vi "数据查询_仪器数据.vi"() -> ()   [LabVIEW 2016, in "数据查询.lvlib"]
uses:
  <vilib>/Utility/miscctls.llb/LVPointTypeDef.ctl
  <vilib>/Utility/miscctls.llb/LVDateTimeRec.ctl
  <vilib>/Utility/miscctls.llb/LVRowAndColumnUnsignedTypeDef.ctl
  <userlib>/_OpenG.lib/array/array.llb/Sort 2D Array (String)__ogtk.vi
  <vilib>/ptbypt/NI_PtbyPt.lvlib
panel:
  out "技术要求":T1={"氨氮"=[0.2, 0.05, 0.1, 0.1], "总磷"=[0.02, 0.05, 0.1, 0.1], "总氮"=[0.3, 0.05, 0.1, 0.1], "CODMn"=[1.5, 0.1, 0.1, 0.1], "CODCr"=[5.0, 0.05, 0.1, 0.1]}
  in  "技术要求":bool
  in  "参数选择":string(combo)="全部数据"
  out "布尔":bool=TRUE
  in  "显示关键参数":bool
  in  "剔除异常数据":bool
  in  "数据类型":string(combo)="全部数据"
  in  "列表框":i32(listbox)
  in  "页":i32 format="第%.0f页"
  in  "每页条数":i32=1000
  in  "向后按钮":bool
  in  "向前按钮":bool
  in  "导出":bool
  in  "测量模式":string(combo)="全部数据"
  in  "查询":bool
  in  "结束日期":string="2050/01/01"
  in  "起始日期":string="2010/01/01"
  out "数据表":string[][](table)
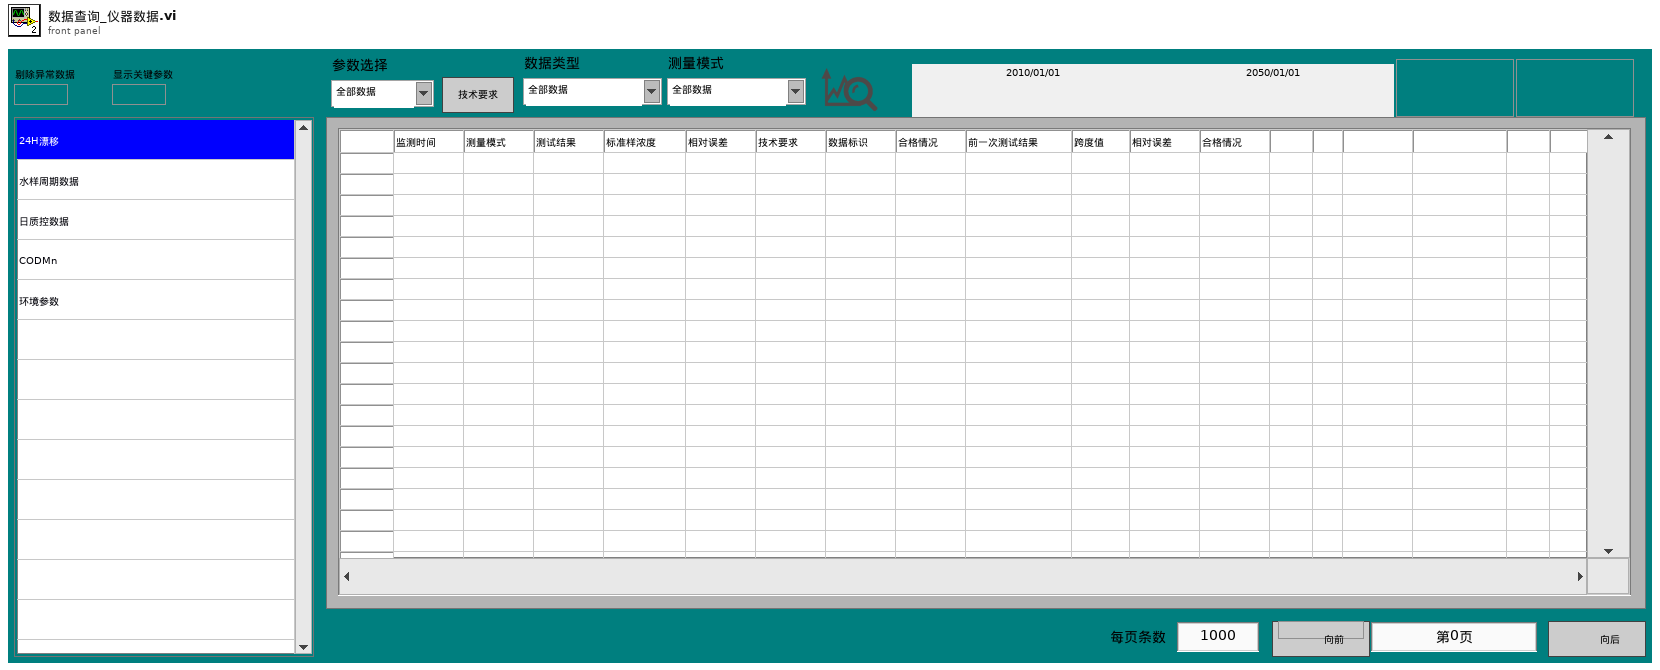
[diagram p1: front panel]
types:
  T1 = cluster{"氨氮":dbl[], "总磷":dbl[], "总氮":dbl[], "CODMn":dbl[], "CODCr":dbl[]}
  T2 = typedef "LVPointTypeDef.ctl" = cluster{"Horizontal":i16, "Vertical":i16}
  T3 = typedef "LVDateTimeRec.ctl" = cluster{"秒数的小数部分":dbl, "秒":i32, "分":i32, "时":i32, "日":i32, "月":i32, "年":i32, "天数（周）":i32, "天数（年）":i32, "DST":i32}
  T4 = typedef "Rendezvous RefNum" = refnum<k1>
  T5 = typedef "数据查询.lvlib/数据查询单选控件.ctl" = enum32{"数据查询", "仪器数据", "仪器日志", "报警信息", "校准日志"}
  T6 = enum8{"Enabled", "Disabled", "Disabled and Grayed Out"}
  T7 = cluster{"索引起始时间":timestamp, "索引终止时间":timestamp, "模式":enum16{"零点核查", "跨度核查"}, "table":string, "误差":enum16{"绝对误差", "相对误差"}, "技术要求":sgl, "24H漂移技术要求":sgl}
  T8 = typedef "LVRowAndColumnUnsignedTypeDef.ctl" = cluster{"Row":u32, "Column":u32}
  T9 = typedef "数据库类型.ctl" = enum16{"Access", "SQLite"}
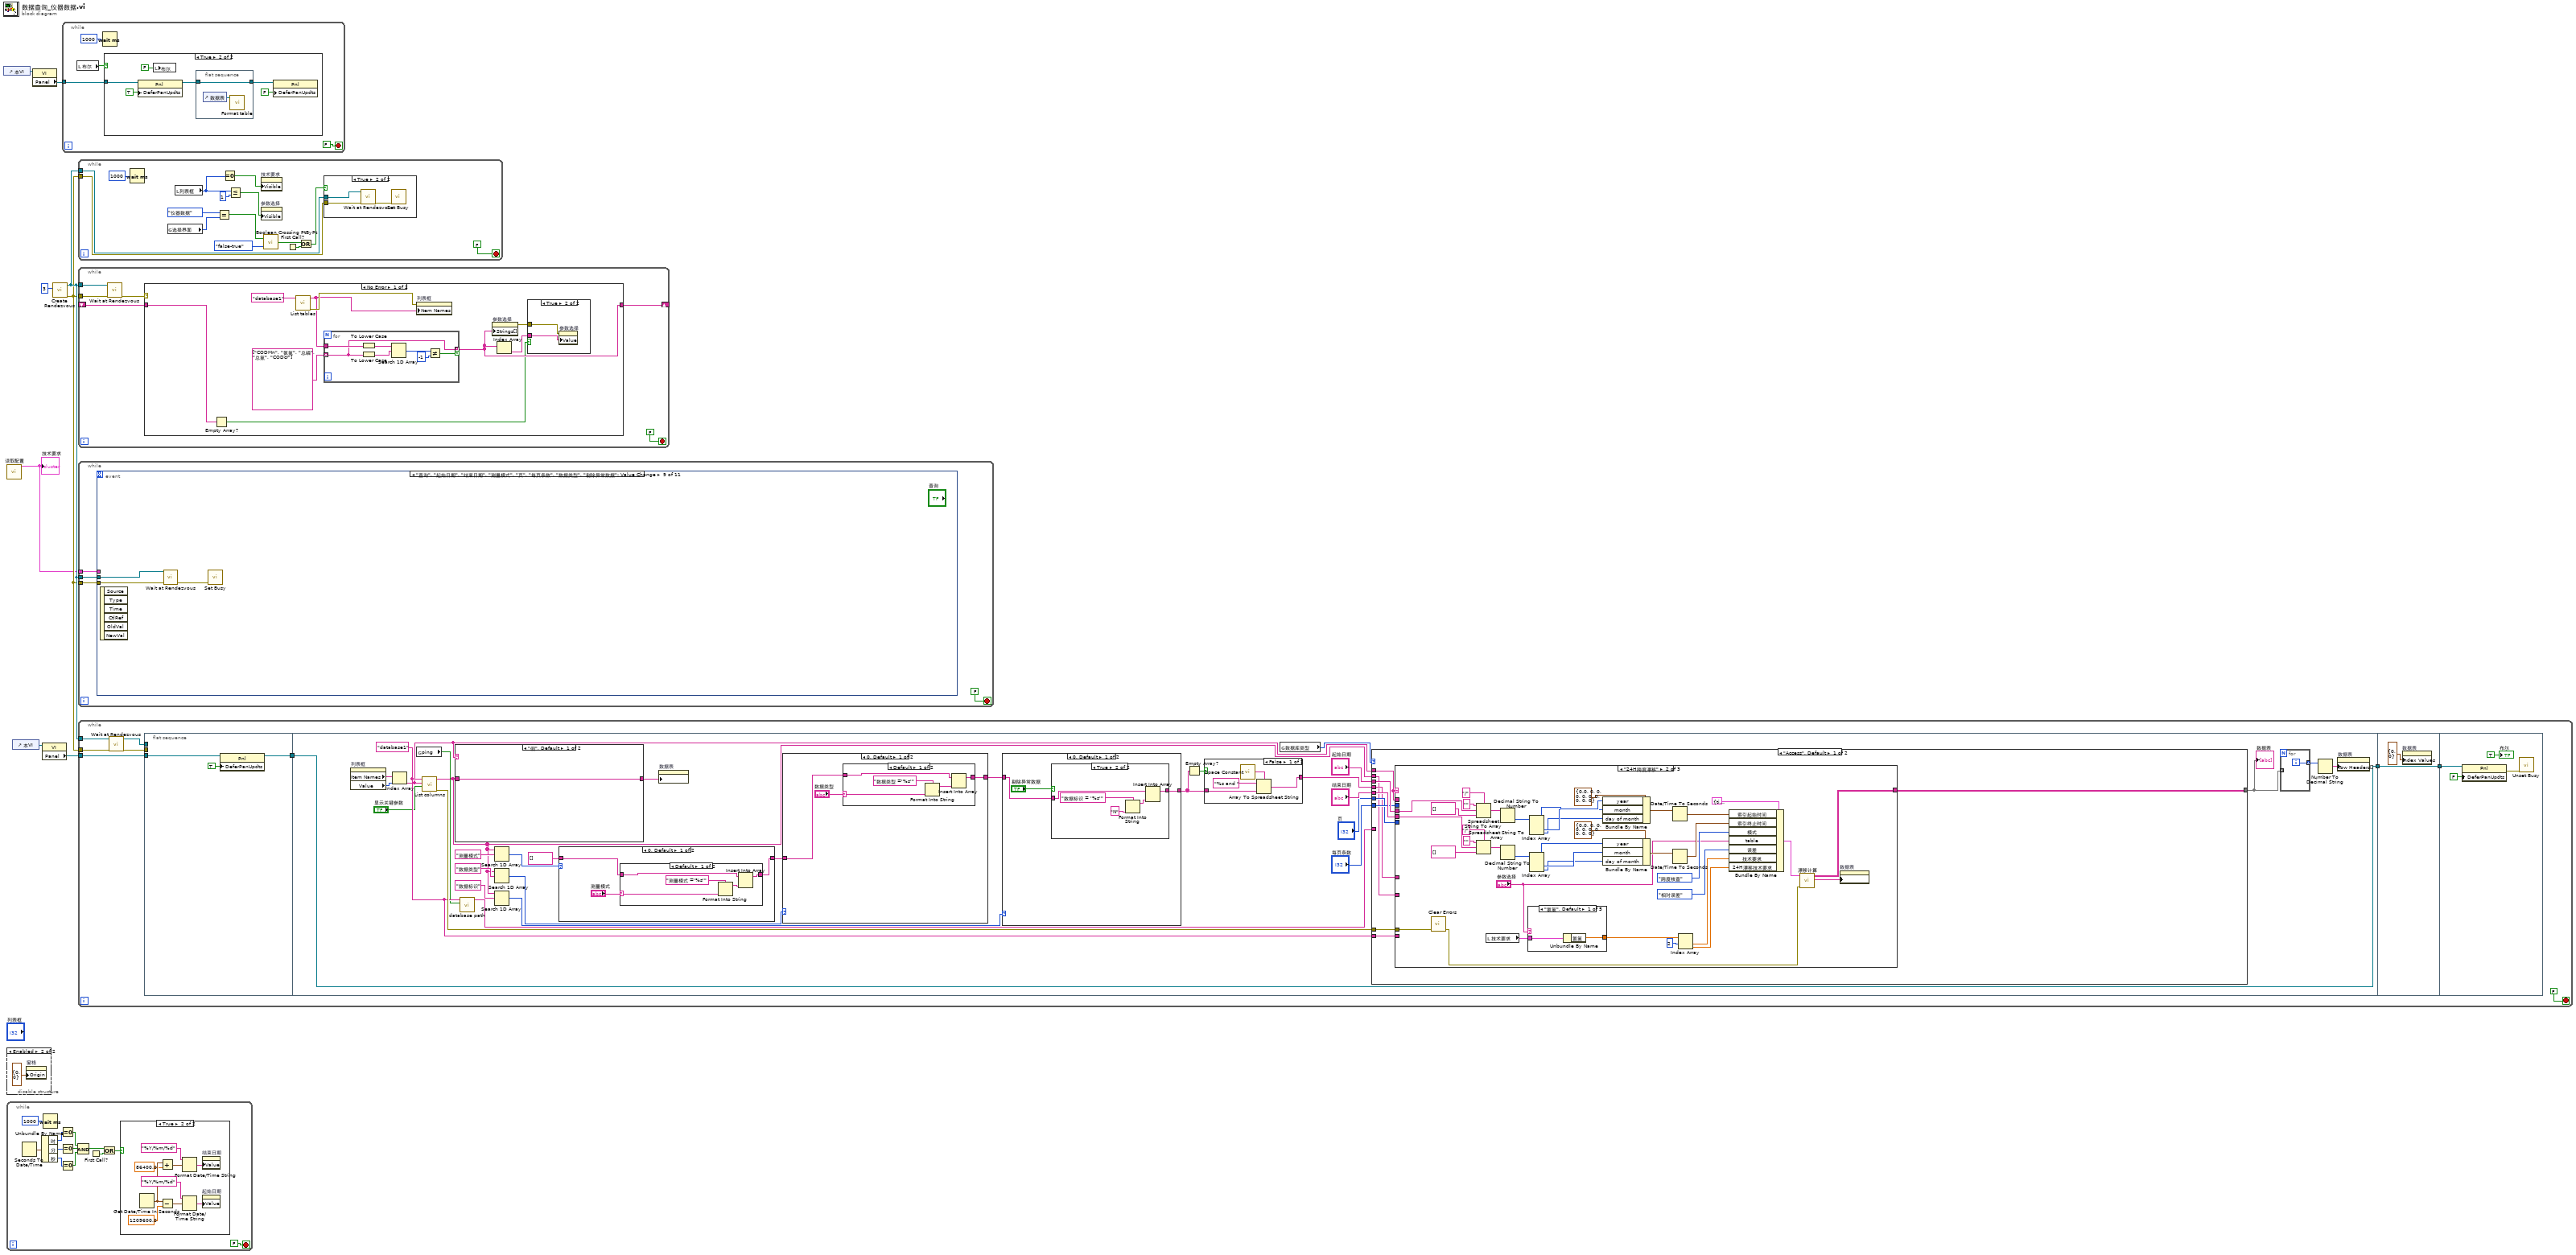
[diagram p0: block diagram]
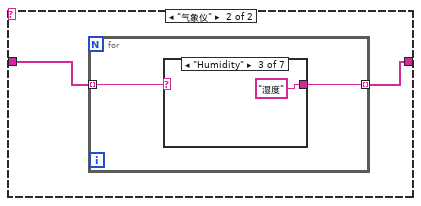
[diagram p6: hidden frame]
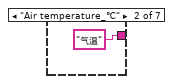
[diagram p8: hidden frame]
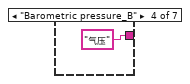
[diagram p9: hidden frame]
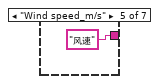
[diagram p10: hidden frame]
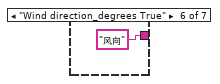
[diagram p11: hidden frame]
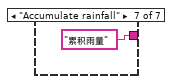
[diagram p12: hidden frame]
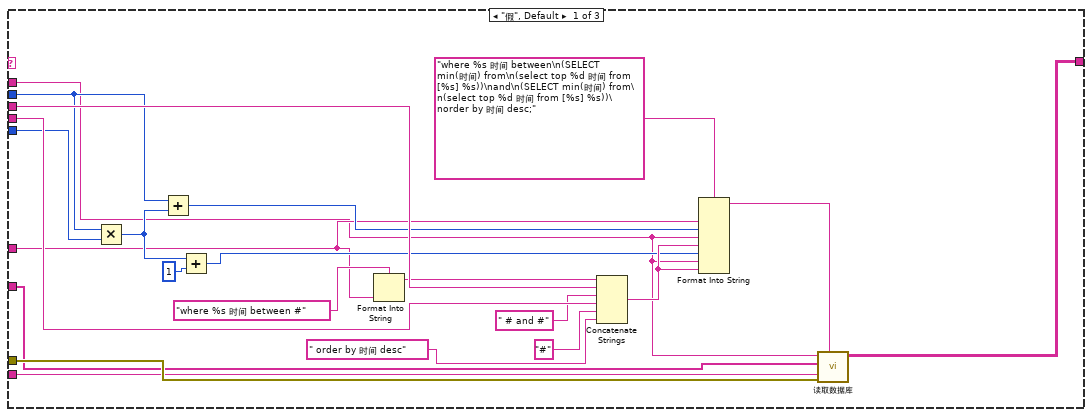
[diagram p13: hidden frame]
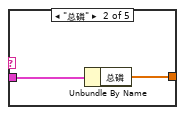
[diagram p14: hidden frame]
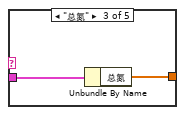
[diagram p15: hidden frame]
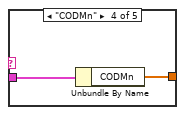
[diagram p16: hidden frame]
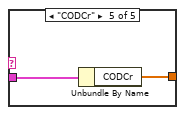
[diagram p17: hidden frame]
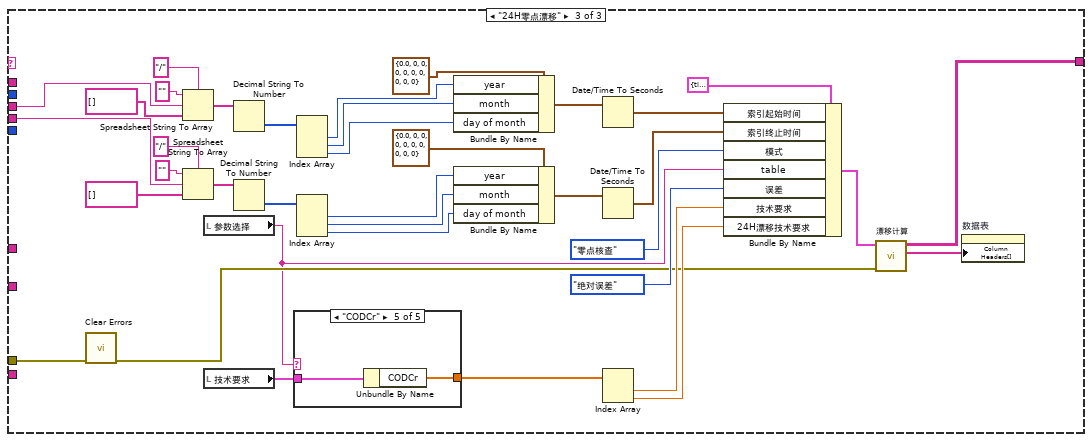
[diagram p18: hidden frame]
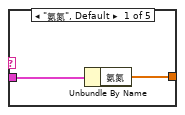
[diagram p19: hidden frame]
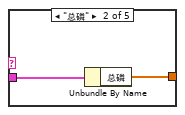
[diagram p20: hidden frame]
diagram:
  n1 = control-ref of="本VI"() -> (w5:refnum<vi>)
  n2 = call "读取配置.vi"() -> ("输入簇"=w1:T1)  [unwired: 11 in]
  "技术要求" <- w1
  n3 = disable-structure shown="Enabled" {
    frame Disabled {
    }
    frame Enabled {
      n4 = property on="窗格" class="Pane"("Origin"=T2 {"Horizontal"=0, "Vertical"=0} ("原点")) -> ()  [unwired: 2 in, 2 out]
    }
  }
  n5 = while {
    stop <- FALSE stop-if-true
    n6 = Seconds To Date/Time() -> (date time rec=w21:T3)  [unwired: 2 in]
    n7 = Unbundle By Name(w21) -> ("时"=w20:i32, "分"=w19:i32, "秒"=w18:i32)
    n8 = Wait (ms)(milliseconds to wait=u32 1000 ("等待时间（毫秒）")) -> ()  [unwired: 1 out]
    n9 = Equal To 0?(x=w20) -> (x = 0?=w17:bool)
    n10 = Equal To 0?(x=w19) -> (x = 0?=w16:bool)
    n11 = Equal To 0?(x=w18) -> (x = 0?=w15:bool)
    n12 = Compound Arithmetic op=AND ("复合运算")(w17, w16, w15) -> (w12:bool)
    n13 = First Call?() -> (First Call?: T/F=w11:bool)
    n14 = Or(x=w12, y=w11) -> (x .or. y?=w10:bool)
    n15 = case shown="True" w10 {
      frame False {
      }
      frame True {
        n16 = Get Date/Time In Seconds() -> (seconds since 1Jan1904=w26:timestamp)
        n17 = Add(x=w26, y=86400.0) -> (x+y=w24:timestamp)
        n18 = Subtract(x=w26, y=1209600.0) -> (x-y=w27:timestamp)
        n19 = Format Date/Time String(time format string (%c)="%Y/%m/%d" ("时间格式字符串(%c)"), seconds (now)=w24) -> (date/time string=w23:string)  [unwired: 1 in]
        n20 = Format Date/Time String(time format string (%c)="%Y/%m/%d" ("时间格式字符串(%c)"), seconds (now)=w27) -> (date/time string=w29:string)  [unwired: 1 in]
        n21 = property on="结束日期" class="Str"("Value"=w23) -> ()  [unwired: 2 in, 2 out]
        n22 = property on="起始日期" class="Str"("Value"=w29) -> ()  [unwired: 2 in, 2 out]
      }
    }
  }
  n23 = control-ref of="本VI"() -> (w8:refnum<vi>)
  n24 = property class="VI"(reference=w5) -> ("Panel"=w4:refnum<vi>)  [unwired: 1 in, 2 out]
  n25 = property class="VI"(reference=w8) -> ("Panel"=w7:refnum<vi>)  [unwired: 1 in, 2 out]
  n26 = call <vilib>:"Create Rendezvous.vi"("size (2)"=3) -> ("error out"=w2:errorcluster, "rendezvous"=w3:T4)  [unwired: 4 in, 1 out]
  n27 = while {
    tunnel: w4 -> [w33]
    stop <- FALSE stop-if-true
    n28 = local read "布尔"() -> (w32:bool)
    n29 = Wait (ms)(milliseconds to wait=u32 1000 ("等待时间（毫秒）")) -> ()  [unwired: 1 out]
    n30 = case shown="True" w32 {
      tunnel: w33 -> [_ w39]
      frame False {
      }
      frame True {
        n31 = property class="Pnl"(reference=w39, "DeferPanUpdts"=TRUE ("延迟前面板更新")) -> (reference out=w38:refnum<vi>)  [unwired: 1 in, 1 out]
        n32 = local write "布尔"(FALSE ("布尔")) -> ()
        n33 = flat-sequence {
          tunnel: [w42] -> w37
          tunnel: w38 -> [w42]
          frame #0 {
            n34 = control-ref of="数据表"() -> (w41:refnum<vi>)
            n35 = call "Format table.vi"("Table输入"=w41) -> ()  [unwired: 11 in]
          }
        }
        n36 = property class="Pnl"(reference=w37, "DeferPanUpdts"=FALSE ("延迟前面板更新")) -> ()  [unwired: 1 in, 2 out]
      }
    }
  }
  n37 = while {
    tunnel: w3 -> [w48]
    tunnel: w2 -> [w47]
    stop <- FALSE stop-if-true
    n38 = Wait (ms)(milliseconds to wait=u32 1000 ("等待时间（毫秒）")) -> ()  [unwired: 1 out]
    n39 = global read "全局变量.vi" "选择界面"() -> (w55:T5)
    n40 = local read "列表框"() -> (w45:i32)
    n41 = Equal?(x=数据查询单选控件."仪器数据", y=w55) -> (x = y?=w53:bool)
    n42 = Equal To 0?(x=w45) -> (x = 0?=w46:bool)
    n43 = Less Or Equal?(x=w45, y=1) -> (x <= y?=w43:bool)
    n44 = property on="技术要求" class="Bool"("Visible"=w46) -> ()  [unwired: 2 in, 2 out]
    n45 = property on="参数选择" class="CmbBox"("Visible"=w43) -> ()  [unwired: 2 in, 2 out]
    n46 = call <vilib>:"Boolean Crossing PtByPt.vi"("direction"=enum16{"either", "false-true", "true-false"}."false-true", "input"=w53) -> ("crossing"=w51:bool)  [unwired: 1 in]
    n47 = First Call?() -> (First Call?: T/F=w49:bool)
    n48 = Or(x=w51, y=w49) -> (x .or. y?=w50:bool)
    n49 = case shown="True" w50 {
      tunnel: w48 -> [_ w60]
      tunnel: w47 -> [_ w59]
      frame False {
      }
      frame True {
        n50 = call <vilib>:"Wait at Rendezvous.vi"("error in (no error)"=w59, "rendezvous"=w60) -> ("error out"=w58:errorcluster)  [unwired: 3 in, 2 out]
        n51 = call <vilib>:"Set Busy.vi"("error in (no error)"=w58) -> ()  [unwired: 9 in, 2 out]
      }
    }
  }
  n52 = while {
    tunnel: w3 -> [w65]
    tunnel: w2 -> [w64]
    shift-right: [w62] -> _
    shift-left: _ -> [w61]
    stop <- FALSE stop-if-true
    n53 = call <vilib>:"Wait at Rendezvous.vi"("error in (no error)"=w64, "rendezvous"=w65) -> ("error out"=w63:errorcluster)  [unwired: 3 in, 2 out]
    n54 = case shown="No Error" w63 {
      tunnel: [w72 w85] -> w62
      tunnel: w61 -> [w71 w85]
      frame No Error {
        n55 = Empty Array?(array=w71) -> (empty?=w70:bool)
        n56 = call "List tables.vi"("database"="database1") -> ("error out"=w75:errorcluster, "tables"=w67:string[])  [unwired: 9 in]
        n57 = for {
          tunnel: string[] ["CODMn", "氨氮", "总磷", "总氮", "CODcr"] -> [w81] mode=indexing
          tunnel: w67 -> [w84]
          tunnel: [w81] -> w72 mode=indexing if=w78
          n58 = To Lower Case(string=w84) -> (all lower case string=w80:string[])
          n59 = To Lower Case(string=w81) -> (all lower case string=w79:string)
          n60 = Search 1D Array(1D array=w80, element=w79) -> (index of element=w83:i32)  [unwired: 1 in]
          n61 = Not Equal?(x=w83, y=-1 ("x")) -> (x != y?=w78:bool)
        }
        n62 = property on="列表框" class="LstBox (strict)"(error in=w75, "Item Names"=w67) -> ()  [unwired: 1 in, 2 out]
        n63 = property on="参数选择" class="CmbBox"("Strings[]"=w72) -> (error out=w69:errorcluster)  [unwired: 2 in, 1 out]
        n64 = Index Array(array=w72) -> (element=w68:string)  [unwired: 1 in]
        n65 = case shown="True" w70 {
          tunnel: w69 -> [_ w77]
          tunnel: w68 -> [_ w76]
          frame False {
          }
          frame True {
            n66 = property on="参数选择" class="CmbBox"(error in=w77, "Value"=w76) -> ()  [unwired: 1 in, 2 out]
          }
        }
      }
      frame Error {
      }
    }
  }
  n67 = while {
    tunnel: w3 -> [w88]
    tunnel: w2 -> [w87]
    tunnel: w1 -> [w86]
    stop <- FALSE stop-if-true
    n68 = event shown="[8] \"查询\", \"起始日期\", \"结束日期\", \"测量模式\", \"页\", \"每页条数\", \"数据类型\", \"剔除异常数据\": Value Change" {
      selector: _ -> [_ _ _ _ _ _ _ _ _ _ _]
      dyn-events: _ -> [_ _ _ _ _ _ _ _ _ _ _]
      timeout: _ -> [_ _ _ _ _ _ _ _ _ _ _]
      tunnel: w88 -> [_ _ _ _ _ _ _ _ w157 _ w163]
      tunnel: w87 -> [_ _ _ _ _ _ _ _ w156 _ w160]
      tunnel: w86 -> [_ _ _ _ _ _ _ _ _ w159 _]
      event Timeout {
        n69 = event-data() -> ()  [unwired: 1 in, 3 out]
      }
      event "查询": Mouse Down {
        n70 = event-data() -> ()  [unwired: 1 in, 8 out]
        n71 = property on="页" class="DigNum (strict)"("Value"=0 ("页")) -> ()  [unwired: 2 in, 2 out]
      }
      event "每页条数": Mouse Down {
        n72 = event-data() -> ("CtlRef"=w92:refnum<vi>)  [unwired: 1 in, 7 out]
        n73 = property class="DigNum (strict)"(reference=w92) -> (reference out=w93:refnum<vi>, "Value"=w95:i32)  [unwired: 1 in, 1 out]
        n74 = property on="页" class="DigNum (strict)"("Value"=0 ("页")) -> ()  [unwired: 2 in, 2 out]
        n75 = call "数字键盘.vi"("OldNumber"=w95) -> ("NewNumber"=w94:sgl)
        n76 = property class="DigNum (strict)"(reference=w93, "Val(Sgnl)"=w94) -> ()  [unwired: 1 in, 2 out]
      }
      event "页": Mouse Down {
        n77 = event-data() -> ("CtlRef"=w96:refnum<vi>)  [unwired: 1 in, 7 out]
        n78 = property class="DigNum (strict)"(reference=w96) -> (reference out=w97:refnum<vi>, "Value"=w99:i32)  [unwired: 1 in, 1 out]
        n79 = call "数字键盘.vi"("OldNumber"=w99) -> ("NewNumber"=w98:sgl)
        n80 = property class="DigNum (strict)"(reference=w97, "Val(Sgnl)"=w98) -> ()  [unwired: 1 in, 2 out]
      }
      event "向前按钮": Value Change {
        n81 = event-data() -> ()  [unwired: 1 in, 6 out]
        n82 = property on="页" class="DigNum (strict)"() -> ("Value"=w105:i32)  [unwired: 2 in, 2 out]
        n83 = Decrement(x=w105) -> (x-1=w104:i32)
        n84 = In Range and Coerce(upper limit=9999 ("上限"), x=w104, lower limit=0 ("下限")) -> (coerced(x)=w101:i32, In Range?=w100:bool)
        n85 = case shown="True" w100 {
          tunnel: w101 -> [_ w106]
          frame False {
          }
          frame True {
            n86 = property on="页" class="DigNum (strict)"("Val(Sgnl)"=w106) -> ()  [unwired: 2 in, 2 out]
          }
        }
      }
      event "向后按钮": Value Change {
        n87 = event-data() -> ()  [unwired: 1 in, 6 out]
        n88 = property on="页" class="DigNum (strict)"() -> ("Value"=w111:i32)  [unwired: 2 in, 2 out]
        n89 = Increment(x=w111) -> (x+1=w110:i32)
        n90 = In Range and Coerce(upper limit=u32 9999 ("上限"), x=w110, lower limit=u32 0 ("下限")) -> (coerced(x)=w107:u32)  [unwired: 1 out]
        n91 = property on="页" class="DigNum (strict)"("Val(Sgnl)"=w107) -> ()  [unwired: 2 in, 2 out]
      }
      event "导出": Value Change {
        n92 = event-data() -> ("CtlRef"=w112:refnum<vi>)  [unwired: 1 in, 5 out]
        n93 = property class="Bool"(reference=w112, "DisabledEnum"=T6."Disabled and Grayed Out" ("禁用")) -> (reference out=w116:refnum<vi>, error out=w117:errorcluster)  [unwired: 1 in]
        n94 = flat-sequence {
          tunnel: w117 -> [_]
          tunnel: [w136] -> w115
          tunnel: w116 -> [w136]
          tunnel: "导出" -> [_]
          frame #0 {
            n95 = local read "数据表"() -> (w140:string[][])
            n96 = call-poly <userlib>:"Sort Array__ogtk.vi"("Column/Row to Sort By"=u32 0, "Sort By in"=enum16{"row", "column"}."column", "Order"=enum16{"ascending", "descending"}."ascending", "Array in"=w140) -> ("Sorted Array out"=w122:string[][])  [unwired: 4 in, 3 out]
            n97 = for {
              tunnel: w122 -> [w149] mode=indexing
              tunnel: [w148] -> w126 mode=indexing
              i -> [w150]
              n98 = Increment(x=w150) -> (x+1=w146:i32)
              n99 = Number To Decimal String(number=w146) -> (decimal integer string=w145:string)  [unwired: 1 in]
              n100 = Insert Into Array(array=w149, index=0 ("索引"), new element=w145) -> (w148:string[])
            }
            n101 = property on="数据表" class="Tbl (strict)"() -> ("Column Headers[]"=w129:string[])  [unwired: 2 in, 2 out]
            n102 = property on="列表框" class="LstBox (strict)"() -> ("Item Names"=w121:string[], "Value"=w120:i32)  [unwired: 2 in, 2 out]
            n103 = Insert Into Array(array=w129, index=0 ("索引"), new element="序号" ("新元素/子数组")) -> (w130:string[])
            n104 = Index Array(array=w121, index=w120) -> (element=w119:string)
            n105 = Format Date/Time String(time format string (%c)="%y_%m_%d" ("时间格式字符串(%c)")) -> (date/time string=w133:string)  [unwired: 2 in]
            n106 = Concatenate Strings(w119, "_" ("字符串"), w133) -> (w131:string)
            n107 = Insert Into Array(array=string[][] [], new element #1=w130, new element #2=w126) -> (w125:string[][])  [unwired: 2 in]
            n108 = call "数据导出Excel.vi"("text data"=w125, "default name"=w131) -> ("error out"=w124:errorcluster, "布尔"=w123:bool)  [unwired: 8 in]
            n109 = case shown="True" w123 {
              tunnel: w124 -> [_ w142]
              frame False {
              }
              frame True {
                n110 = case shown="Error" w142 {
                  tunnel: ["导出成功" ("消息") "导出失败" ("消息")] -> w141
                  frame No Error {
                  }
                  frame Error {
                  }
                }
                n111 = One Button Dialog(message=w141) -> ()  [unwired: 1 in, 1 out]
              }
            }
          }
        }
        n112 = property class="Bool"(reference=w115, "DisabledEnum"=T6."Enabled" ("禁用")) -> ()  [unwired: 1 in, 2 out]
      }
      event "起始日期", "结束日期": Mouse Down {
        n113 = event-data() -> ("CtlRef"=w154:refnum<vi>)  [unwired: 1 in, 7 out]
        n114 = property class="Str"(reference=w154) -> (reference out=w152:refnum<vi>, "Value"=w153:string)  [unwired: 1 in, 1 out]
        n115 = call "日期键盘.vi"("原值"=w153) -> ("x+y"=w151:string)  [unwired: 10 in]
        n116 = property class="Str"(reference=w152, "Val(Sgnl)"=w151) -> ()  [unwired: 1 in, 2 out]
      }
      event "查询", "起始日期", "结束日期", "测量模式", "页", "每页条数", "数据类型", "剔除异常数据": Value Change {
        n117 = event-data() -> ()  [unwired: 1 in, 6 out]
        n118 = call <vilib>:"Wait at Rendezvous.vi"("error in (no error)"=w156, "rendezvous"=w157) -> ("error out"=w155:errorcluster)  [unwired: 3 in, 2 out]
        n119 = call <vilib>:"Set Busy.vi"("error in (no error)"=w155) -> ()  [unwired: 9 in, 2 out]
      }
      event "技术要求": Value Change {
        n120 = event-data() -> ()  [unwired: 1 in, 6 out]
        n121 = call "漂移技术参数设置.vi"("输入簇"=w159) -> ("输出簇"=w158:T1)  [unwired: 10 in]
        n122 = local write "技术要求"(w158) -> ()
      }
      event "列表框": Value Change {
        n123 = event-data() -> ()  [unwired: 1 in, 6 out]
        n124 = flat-sequence {
          tunnel: w163 -> [w167]
          tunnel: [w167] -> w162
          tunnel: [w164] -> w161
          tunnel: w160 -> [w164]
          tunnel: w162 -> [w170]
          tunnel: w161 -> [w169]
          frame #0 {
            n125 = property on="数据类型" class="CmbBox"("Value"="全部数据" ("数据类型")) -> ()  [unwired: 2 in, 2 out]
            n126 = property on="测量模式" class="CmbBox"("Value"="全部数据" ("测量模式")) -> ()  [unwired: 2 in, 2 out]
          }
          frame #1 {
            n127 = call <vilib>:"Wait at Rendezvous.vi"("error in (no error)"=w169, "rendezvous"=w170) -> ("error out"=w168:errorcluster)  [unwired: 3 in, 2 out]
            n128 = call <vilib>:"Set Busy.vi"("error in (no error)"=w168) -> ()  [unwired: 9 in, 2 out]
          }
        }
      }
    }
  }
  n129 = while {
    tunnel: w3 -> [w174]
    tunnel: w7 -> [w178]
    tunnel: w2 -> [w173]
    stop <- FALSE stop-if-true
    n130 = call <vilib>:"Wait at Rendezvous.vi"("error in (no error)"=w173, "rendezvous"=w174) -> ("error out"=w171:errorcluster, "rendezvous out"=w172:T4)  [unwired: 3 in, 1 out]
    n131 = flat-sequence {
      tunnel: w178 -> [w182]
      tunnel: [w180] -> w177
      tunnel: w172 -> [_]
      tunnel: w171 -> [_]
      tunnel: w177 -> [w183]
      tunnel: [w183] -> w175
      tunnel: [w441] -> w176
      tunnel: w175 -> [w441]
      tunnel: w176 -> [w446]
      frame #0 {
        n132 = property class="Pnl"(reference=w182, "DeferPanUpdts"=TRUE ("延迟前面板更新")) -> (reference out=w180:refnum<vi>)  [unwired: 1 in, 1 out]
      }
      frame #1 {
        w191 = "database1" ("database")
        n133 = property on="列表框" class="LstBox (strict)"() -> ("Item Names"=w202:string[], "Value"=w207:i32)  [unwired: 2 in, 2 out]
        n134 = Index Array(array=w202, index=w207) -> (element=w186:string)
        n135 = global read "全局变量.vi" "ping"() -> (w189:bool)
        n136 = call "List columns.vi"("显示关键参数"="显示关键参数", "table"=w186, "database"=w191) -> ("error out"=w201:errorcluster, "columns"=w187:string[])  [unwired: 7 in]
        n137 = case shown="\"假\", Default" w186 {
          tunnel: w187 -> [w214 w216]
          tunnel: [w214 w215] -> w185
          frame "假", Default {
          }
          frame "气象仪" {
            n138 = for {
              tunnel: w216 -> [w218] mode=indexing
              tunnel: [w217] -> w215 mode=indexing
              n139 = case shown="\"Humidity\"" w218 {
                selector: w218 -> [w219 _ _ _ _ _ _]
                tunnel: [w219 "气温" "湿度" "气压" "风速" "风向" "累积雨量"] -> w217
                frame "", Default {
                }
                frame "Air temperature_℃" {
                }
                frame "Humidity" {
                }
                frame "Barometric pressure_B" {
                }
                frame "Wind speed_m/s" {
                }
                frame "Wind direction_degrees True" {
                }
                frame "Accumulate rainfall" {
                }
              }
            }
          }
        }
        n140 = call "database path.vi"("ping"=w189, "database"=w191) -> ("Path out"=w190:string)  [unwired: 8 in, 1 out]
        n141 = Search 1D Array(1D array=w187, element="测量模式" ("元素")) -> (index of element=w195:i32)  [unwired: 1 in]
        n142 = Search 1D Array(1D array=w187, element="数据类型" ("元素")) -> (index of element=w198:i32)  [unwired: 1 in]
        n143 = Search 1D Array(1D array=w187, element="数据标识" ("元素")) -> (index of element=w196:i32)  [unwired: 1 in]
        n144 = case shown="0, Default" w195 {
          tunnel: string[] [] -> [w412 w419]
          tunnel: [w410 w419] -> w204
          frame 0, Default {
            n145 = case shown="Default" "测量模式" {
              selector: "测量模式" -> [w413 _]
              tunnel: w412 -> [w416 w418]
              tunnel: [w414 w418] -> w410
              frame Default {
                n146 = Format Into String(format string="测量模式 ='%s'" ("condition"), w413) -> (resulting string=w415:string)  [unwired: 2 in, 1 out]
                n147 = Insert Into Array(array=w416, new element=w415) -> (w414:string[])  [unwired: 1 in]
              }
              frame "全部数据" {
              }
            }
          }
          frame -1 {
          }
        }
        n148 = property on="数据表" class="Tbl (strict)"("Column Headers[]"=w185) -> ()  [unwired: 2 in, 2 out]
        n149 = case shown="0, Default" w198 {
          tunnel: w204 -> [w432 w439]
          tunnel: [w431 w439] -> w200
          frame 0, Default {
            n150 = case shown="Default" "数据类型" {
              selector: "数据类型" -> [w433 _]
              tunnel: w432 -> [w436 w438]
              tunnel: [w434 w438] -> w431
              frame Default {
                n151 = Format Into String(format string="数据类型 ='%s'" ("condition"), w433) -> (resulting string=w435:string)  [unwired: 2 in, 1 out]
                n152 = Insert Into Array(array=w436, new element=w435) -> (w434:string[])  [unwired: 1 in]
              }
              frame "全部数据" {
              }
            }
          }
          frame -1 {
          }
        }
        n153 = case shown="0, Default" w196 {
          tunnel: [w422 w429] -> w193
          tunnel: w200 -> [w420 w429]
          frame 0, Default {
            n154 = case shown="True" "剔除异常数据" {
              tunnel: w420 -> [w423 w428]
              tunnel: [w423 w427] -> w422
              frame False {
              }
              frame True {
                n155 = Format Into String(format string="数据标识 = '%s'" ("condition"), "N" ("String")) -> (resulting string=w424:string)  [unwired: 2 in, 1 out]
                n156 = Insert Into Array(array=w428, new element=w424) -> (w427:string[])  [unwired: 1 in]
              }
            }
          }
          frame -1 {
          }
        }
        n157 = Empty Array?(array=w193) -> (empty?=w192:bool)
        n158 = case shown="False" w192 {
          tunnel: [w406 "" ("spreadsheet string")] -> w203
          tunnel: w193 -> [w405 _]
          frame False {
            n159 = call <vilib>:"Space Constant.vi"() -> ("String"=w408:string)
            n160 = Array To Spreadsheet String(delimiter (Tab)=w408, array=w405, 3:"%s and " ("格式字符串")) -> (spreadsheet string=w406:string)
          }
          frame True {
          }
        }
        n161 = global read "外部调用接口全局变量.vi" "数据库类型"() -> (w184:T9)
        n162 = case shown="\"Access\", Default" w184 {
          tunnel: "起始日期" -> [w235 w372]
          tunnel: "结束日期" -> [w234 w371]
          tunnel: "每页条数" -> [w233 w369]
          tunnel: "页" -> [w232 w370]
          tunnel: [w231 w359] -> w206
          tunnel: w203 -> [w230 w373]
          tunnel: w201 -> [w229 w375]
          tunnel: w186 -> [w226 w356]
          tunnel: w191 -> [w228 _]
          tunnel: w187 -> [w227 w353]
          tunnel: w190 -> [_ w354]
          frame "Access", Default {
            n163 = case shown="\"24H跨度漂移\"" w226 {
              tunnel: w235 -> [w257 w280 w327]
              tunnel: w234 -> [w256 w269 w316]
              tunnel: w233 -> [w249 _ _]
              tunnel: w232 -> [w248 _ _]
              tunnel: [w247 w294 w341] -> w231
              tunnel: w230 -> [w240 _ _]
              tunnel: w229 -> [w239 w293 w340]
              tunnel: w226 -> [w238 _ _]
              tunnel: w228 -> [w237 _ _]
              tunnel: w227 -> [w236 _ _]
              frame "假", Default {
                n164 = Multiply(x=w249, y=w248) -> (x*y=w245:i32)
                n165 = Add(x=w249, y=w245) -> (x+y=w243:i32)
                n166 = Add(x=w245, y=u32 1) -> (x+y=w242:u32)
                n167 = Format Into String(format string="where %s 时间 between #" ("condition"), w240) -> (resulting string=w253:string)  [unwired: 2 in, 1 out]
                n168 = Concatenate Strings(w253, w257, " # and #" ("condition"), w256, "#" ("condition"), " order by 时间 desc" ("字符串")) -> (w251:string)
                n169 = Format Into String(format string="where %s 时间 between\n(SELECT min(时间) from\n(select top %d 时间 from [%s] %s))\nand\n(SELECT min(时间) from\n(select top %d 时间 from [%s] %s))\norder by 时间 desc;" ("格式字符串"), w240, w243, w238, w251, w242, w238, w251) -> (resulting string=w250:string)  [unwired: 2 in, 1 out]
                n170 = call "读取数据库.vi"("condition"=w250, "error in (no error)"=w239, "database"=w237, "显示项"=w236, "组合框"=w238) -> ("表格"=w247:string[][])  [unwired: 3 in, 3 out]
              }
              frame "24H跨度漂移" {
                n171 = call <vilib>:"Clear Errors.vi"("error in (no error)"=w293) -> ("error out"=w260:errorcluster)  [unwired: 5 in, 1 out]
                n172 = Spreadsheet String To Array(delimiter (Tab)="/" ("分隔符(Tab)"), format string="" ("格式字符串"), spreadsheet string=w280, array type (2D Dbl)=string[] []) -> (array=w289:string[])
                n173 = Spreadsheet String To Array(delimiter (Tab)="/" ("分隔符(Tab)"), format string="" ("格式字符串"), spreadsheet string=w269, array type (2D Dbl)=string[] []) -> (array=w276:string[])
                n174 = local read "技术要求"() -> (w261:T1)
                n175 = Decimal String To Number(string=w289) -> (number=w288:i32[])  [unwired: 2 in, 1 out]
                n176 = Decimal String To Number(string=w276) -> (number=w275:i32[])  [unwired: 2 in, 1 out]
                n177 = case shown="\"氨氮\", Default" "参数选择" {
                  tunnel: w261 -> [w297 w299 w301 w303 w305]
                  tunnel: [w296 w298 w300 w302 w304] -> w258
                  frame "氨氮", Default {
                    n178 = Unbundle By Name(w297) -> ("氨氮"=w296:dbl[])
                  }
                  frame "总磷" {
                    n179 = Unbundle By Name(w299) -> ("总磷"=w298:dbl[])
                  }
                  frame "总氮" {
                    n180 = Unbundle By Name(w301) -> ("总氮"=w300:dbl[])
                  }
                  frame "CODMn" {
                    n181 = Unbundle By Name(w303) -> ("CODMn"=w302:dbl[])
                  }
                  frame "CODCr" {
                    n182 = Unbundle By Name(w305) -> ("CODCr"=w304:dbl[])
                  }
                }
                n183 = Index Array(array=w288) -> (element #1=w287:i32, element #2=w286:i32, element #3=w285:i32)  [unwired: 3 in]
                n184 = Index Array(array=w275) -> (element #1=w274:i32, element #2=w273:i32, element #3=w272:i32)  [unwired: 3 in]
                n185 = Bundle By Name(cluster=T3 {"fractional second"=0.0, "second"=0, "minute"=0, "hour"=0, "day of month"=0, "month"=0, "year"=0, "day of week"=0, "day of year"=0, "DST"=0} ("日期时间记录"), "year"=w287, "month"=w286, "day of month"=w285) -> (w284:T3)
                n186 = Bundle By Name(cluster=T3 {"fractional second"=0.0, "second"=0, "minute"=0, "hour"=0, "day of month"=0, "month"=0, "year"=0, "day of week"=0, "day of year"=0, "DST"=0} ("日期时间记录"), "year"=w274, "month"=w273, "day of month"=w272) -> (w271:T3)
                n187 = Date/Time To Seconds(2:w284) -> (0:w281:timestamp)  [unwired: 1 in]
                n188 = Date/Time To Seconds(2:w271) -> (0:w268:timestamp)  [unwired: 1 in]
                n189 = Index Array(array=w258, index #1=2 ("索引")) -> (element #1=w264:dbl, element #2=w263:dbl)  [unwired: 1 in]
                n190 = Bundle By Name(cluster=T7 {"索引起始时间"=timestamp(0 s since 1904-01-01), "索引终止时间"=timestamp(0 s since 1904-01-01), "模式"=enum."零点核查", "table"="", "误差"=enum."绝对误差", "技术要求"=0.2, "24H漂移技术要求"=0.05} ("input"), "索引起始时间"=w281, "索引终止时间"=w268, "模式"=enum16{"零点核查", "跨度核查"}."跨度核查", "table"="参数选择", "误差"=enum16{"绝对误差", "相对误差"}."相对误差", "技术要求"=w264, "24H漂移技术要求"=w263) -> (w267:T7)
                n191 = call "漂移计算.vi"("error in (no error)"=w260, "input"=w267) -> ("列首字符串[]"=w295:string[], "表格控件"=w294:string[][])  [unwired: 7 in, 1 out]
                n192 = property on="数据表" class="Tbl (strict)"("Column Headers[]"=w295) -> ()  [unwired: 2 in, 2 out]
              }
              frame "24H零点漂移" {
                n193 = call <vilib>:"Clear Errors.vi"("error in (no error)"=w340) -> ("error out"=w308:errorcluster)  [unwired: 5 in, 1 out]
                n194 = Spreadsheet String To Array(delimiter (Tab)="/" ("分隔符(Tab)"), format string="" ("格式字符串"), spreadsheet string=w327, array type (2D Dbl)=string[] []) -> (array=w336:string[])
                n195 = Spreadsheet String To Array(delimiter (Tab)="/" ("分隔符(Tab)"), format string="" ("格式字符串"), spreadsheet string=w316, array type (2D Dbl)=string[] []) -> (array=w323:string[])
                n196 = local read "参数选择"() -> (w307:string)
                n197 = local read "技术要求"() -> (w309:T1)
                n198 = Decimal String To Number(string=w336) -> (number=w335:i32[])  [unwired: 2 in, 1 out]
                n199 = Decimal String To Number(string=w323) -> (number=w322:i32[])  [unwired: 2 in, 1 out]
                n200 = case shown="\"CODCr\"" w307 {
                  tunnel: w309 -> [w344 w346 w348 w350 w352]
                  tunnel: [w343 w345 w347 w349 w351] -> w306
                  frame "氨氮", Default {
                    n201 = Unbundle By Name(w344) -> ("氨氮"=w343:dbl[])
                  }
                  frame "总磷" {
                    n202 = Unbundle By Name(w346) -> ("总磷"=w345:dbl[])
                  }
                  frame "总氮" {
                    n203 = Unbundle By Name(w348) -> ("总氮"=w347:dbl[])
                  }
                  frame "CODMn" {
                    n204 = Unbundle By Name(w350) -> ("CODMn"=w349:dbl[])
                  }
                  frame "CODCr" {
                    n205 = Unbundle By Name(w352) -> ("CODCr"=w351:dbl[])
                  }
                }
                n206 = Index Array(array=w335) -> (element #1=w334:i32, element #2=w333:i32, element #3=w332:i32)  [unwired: 3 in]
                n207 = Index Array(array=w322) -> (element #1=w321:i32, element #2=w320:i32, element #3=w319:i32)  [unwired: 3 in]
                n208 = Bundle By Name(cluster=T3 {"fractional second"=0.0, "second"=0, "minute"=0, "hour"=0, "day of month"=0, "month"=0, "year"=0, "day of week"=0, "day of year"=0, "DST"=0} ("日期时间记录"), "year"=w334, "month"=w333, "day of month"=w332) -> (w331:T3)
                n209 = Bundle By Name(cluster=T3 {"fractional second"=0.0, "second"=0, "minute"=0, "hour"=0, "day of month"=0, "month"=0, "year"=0, "day of week"=0, "day of year"=0, "DST"=0} ("日期时间记录"), "year"=w321, "month"=w320, "day of month"=w319) -> (w318:T3)
                n210 = Date/Time To Seconds(2:w331) -> (0:w328:timestamp)  [unwired: 1 in]
                n211 = Date/Time To Seconds(2:w318) -> (0:w315:timestamp)  [unwired: 1 in]
                n212 = Index Array(array=w306) -> (element #1=w311:dbl, element #2=w310:dbl)  [unwired: 2 in]
                n213 = Bundle By Name(cluster=T7 {"索引起始时间"=timestamp(0 s since 1904-01-01), "索引终止时间"=timestamp(0 s since 1904-01-01), "模式"=enum."零点核查", "table"="", "误差"=enum."绝对误差", "技术要求"=0.2, "24H漂移技术要求"=0.05} ("input"), "索引起始时间"=w328, "索引终止时间"=w315, "模式"=enum16{"零点核查", "跨度核查"}."零点核查", "table"=w307, "误差"=enum16{"绝对误差", "相对误差"}."绝对误差", "技术要求"=w311, "24H漂移技术要求"=w310) -> (w314:T7)
                n214 = call "漂移计算.vi"("error in (no error)"=w308, "input"=w314) -> ("列首字符串[]"=w342:string[], "表格控件"=w341:string[][])  [unwired: 7 in, 1 out]
                n215 = property on="数据表" class="Tbl (strict)"("Column Headers[]"=w342) -> ()  [unwired: 2 in, 2 out]
              }
            }
          }
          frame "SQLite" {
            n216 = Multiply(x=w369, y=w370) -> (x*y=w368:i32)
            n217 = Format Into String(format string="%s 时间 between '%s' and '%s' order by 时间 desc limit %d,%d" ("格式字符串"), w373, w372, w371, w368, w369) -> (resulting string=w364:string)  [unwired: 2 in, 1 out]
            n218 = Search and Replace String(replace all?=TRUE ("替换全部？(F)"), input string=w364, search string="/" ("搜索字符串"), replace string="-" ("替换字符串(\"\")")) -> (result string=w363:string)  [unwired: 4 in, 3 out]
            n219 = call "精度表.vi"() -> ("精度"=w358:i32[], "参数"=w357:string[])  [unwired: 10 in]
            n220 = call "Select Str.vi"("DB Path"=w354, "Where Clause"=w363, "Tables Name"=w356, "error in (no error)"=w375, "Columns"=w353) -> ("Results"=w362:string[][])  [unwired: 7 in, 3 out]
            n221 = Search 1D Array(1D array=w357, element=w356) -> (index of element=w355:i32)  [unwired: 1 in]
            n222 = Transpose 2D Array(2D array=w362) -> (transposed array=w361:string[][])
            n223 = for {
              tunnel: w353 -> [w377] mode=indexing
              tunnel: w361 -> [w382] mode=indexing
              tunnel: [w381] -> w360 mode=indexing
              tunnel: w356 -> [_]
              tunnel: w357 -> [w378]
              tunnel: w358 -> [w380]
              tunnel: w355 -> [w376]
              n224 = Search 1D Array(1D array=w378, element=w377) -> (index of element=w379:i32)  [unwired: 1 in]
              n225 = case shown="0, Default" w379 {
                selector: w379 -> [w384 _]
                tunnel: w382 -> [w392 w404]
                tunnel: [w391 w404] -> w381
                tunnel: w380 -> [w390 _]
                tunnel: w377 -> [w387 _]
                tunnel: w376 -> [w385 _]
                frame 0, Default {
                  n226 = Equal?(x=w387, y="检测值" ("元素")) -> (x = y?=w386:bool)
                  n227 = Select(t=w385, s=w386, f=w384) -> (s? t:f=w383:i32)
                  n228 = Index Array(array=w390, index=w383) -> (element=w389:i32)
                  n229 = for {
                    tunnel: w392 -> [w394] mode=indexing
                    tunnel: [w395] -> w391 mode=indexing
                    tunnel: w389 -> [w396]
                    n230 = Empty String/Path?(string/path=w394) -> (empty?=w393:bool)
                    n231 = case shown="False" w393 {
                      tunnel: w396 -> [w401 _]
                      tunnel: [w398 w403] -> w395
                      tunnel: w394 -> [w397 w403]
                      frame False {
                        n232 = Fract/Exp String To Number(string=w397) -> (number=w402:dbl)  [unwired: 3 in, 1 out]
                        n233 = Format Into String(format string="%%.%df" ("格式字符串"), w401) -> (resulting string=w400:string)  [unwired: 2 in, 1 out]
                        n234 = Format Into String(format string=w400, w402) -> (resulting string=w398:string)  [unwired: 2 in, 1 out]
                      }
                      frame True {
                      }
                    }
                  }
                }
                frame -1 {
                }
              }
            }
            n235 = Transpose 2D Array(2D array=w360) -> (transposed array=w359:string[][])
          }
        }
        "数据表" <- w206
        n236 = for {
          tunnel: w206 -> [_] mode=indexing
          tunnel: [w440] -> w211 mode=indexing
          i -> [w440]
        }
        n237 = Number To Decimal String(number=w211) -> (decimal integer string=w210:string[])  [unwired: 1 in]
        n238 = property on="数据表" class="Tbl (strict)"("Row Headers[]"=w210) -> ()  [unwired: 2 in, 2 out]
      }
      frame #2 {
        n239 = property on="数据表" class="Tbl (strict)"("Index Values"=T8 {"Row"=0, "Column"=0} ("索引值")) -> ()  [unwired: 2 in, 2 out]
      }
      frame #3 {
        n240 = property class="Pnl"(reference=w446, "DeferPanUpdts"=FALSE ("延迟前面板更新")) -> (error out=w444:errorcluster)  [unwired: 1 in, 1 out]
        n241 = call <vilib>:"Unset Busy.vi"("error in (no error)"=w444) -> ()  [unwired: 10 in, 1 out]
        "布尔" <- TRUE
      }
    }
  }
